vi "LV SciSDK CUSTOM PACKET.vi"(8 "error in (no error)":errorcluster, 9 "CP Handle In":T2) -> (0 "error out":errorcluster, 1 "CP Handle Out":T2, 2 "buffer out":T1, 3 "function return":i32)   [LabVIEW 2021]
uses:
  SciSDK_Labview.lvlib
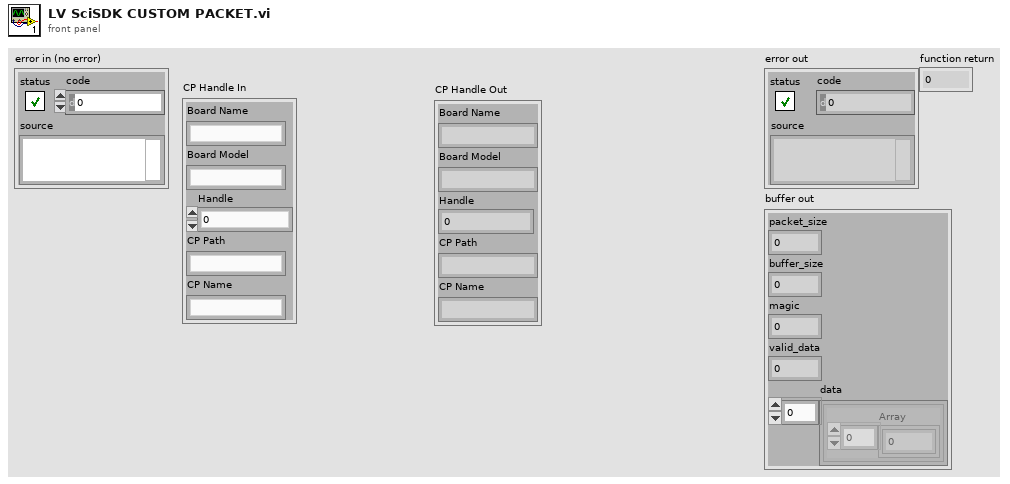
[diagram p1: front panel]
types:
  T1 = cluster{"packet_size":u32, "buffer_size":u32, "magic":u32, "valid_data":dbl, "data":cluster{"Array":dbl[]}[]}
  T2 = cluster{"Board Name":string, "Board Model":string, "Handle":u64, "CP Path":string, "CP Name":string}
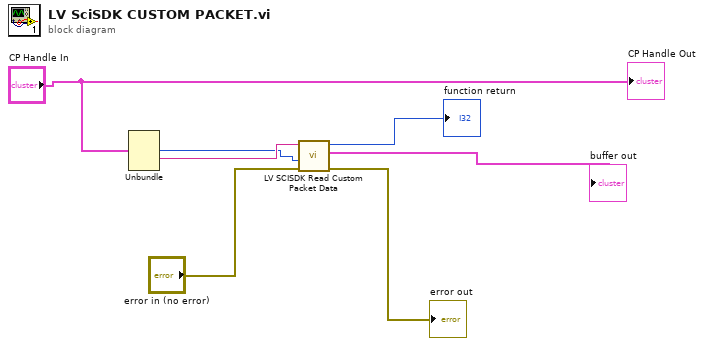
[diagram p0: block diagram]
diagram:
  n1 = Unbundle("CP Handle In") -> ("Handle"=w5:u64, "CP Path"=w6:string)  [unwired: 3 out]
  n2 = call "LV SCISDK Read Custom Packet Data.vi"("Path"=w6, "handle"=w5, "error in (no error)"="error in (no error)") -> ("function return"=→"function return":i32, "buffer out"=→"buffer out":T1, "error out"=→"error out":errorcluster)  [unwired: 4 in, 1 out]
  "CP Handle Out" <- "CP Handle In"
